vi "review.vi"() -> ()   [LabVIEW 2014]
panel:
  out "클러스터 2":T1
  in  "클러스터":T1
  in  "배열":dbl[](array[numeric])
  out "웨이브폼 차트 2":dbl(graph)
  out "웨이브폼 차트":dbl(graph)
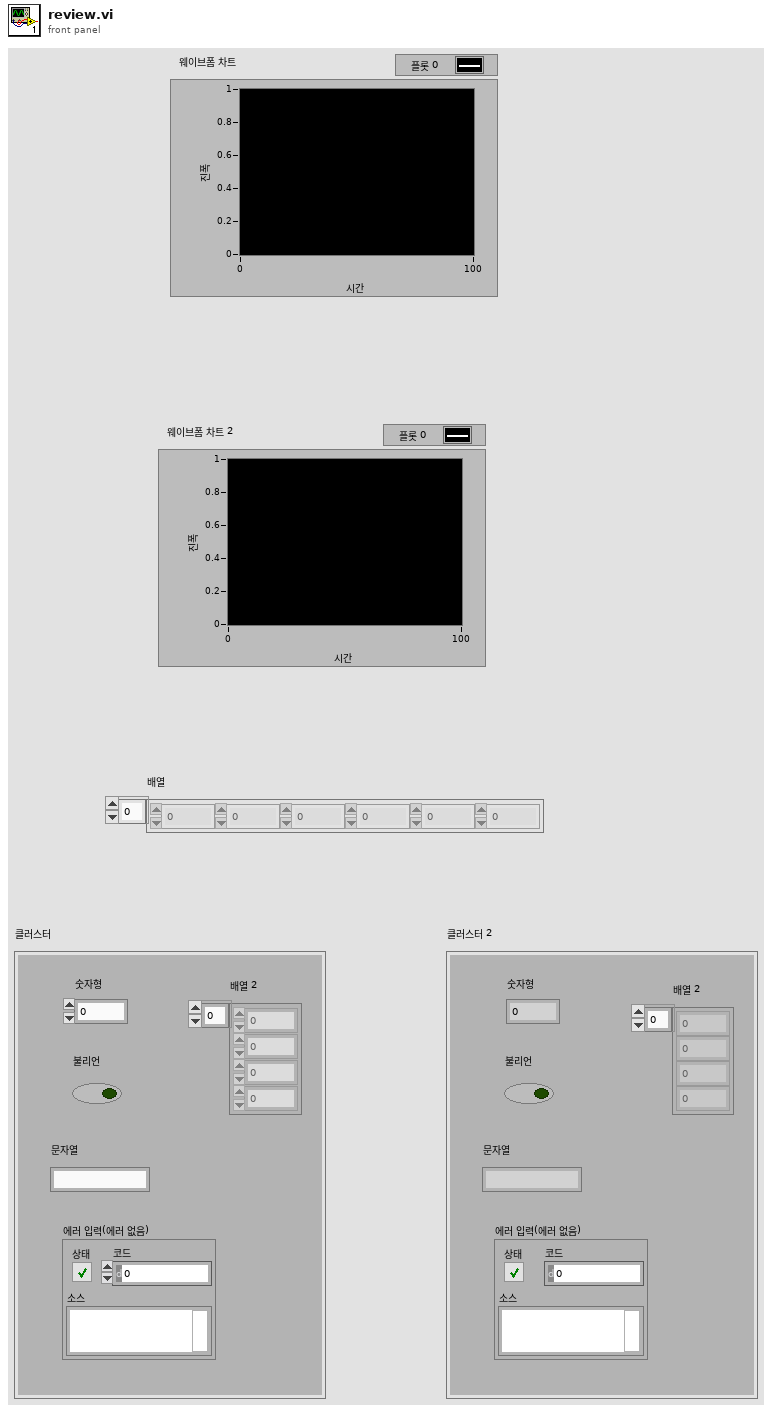
[diagram p1: front panel]
types:
  T1 = cluster{"숫자형":dbl, "불리언":bool, "문자열":string, "배열 2":dbl[], "error in (no error)":errorcluster}
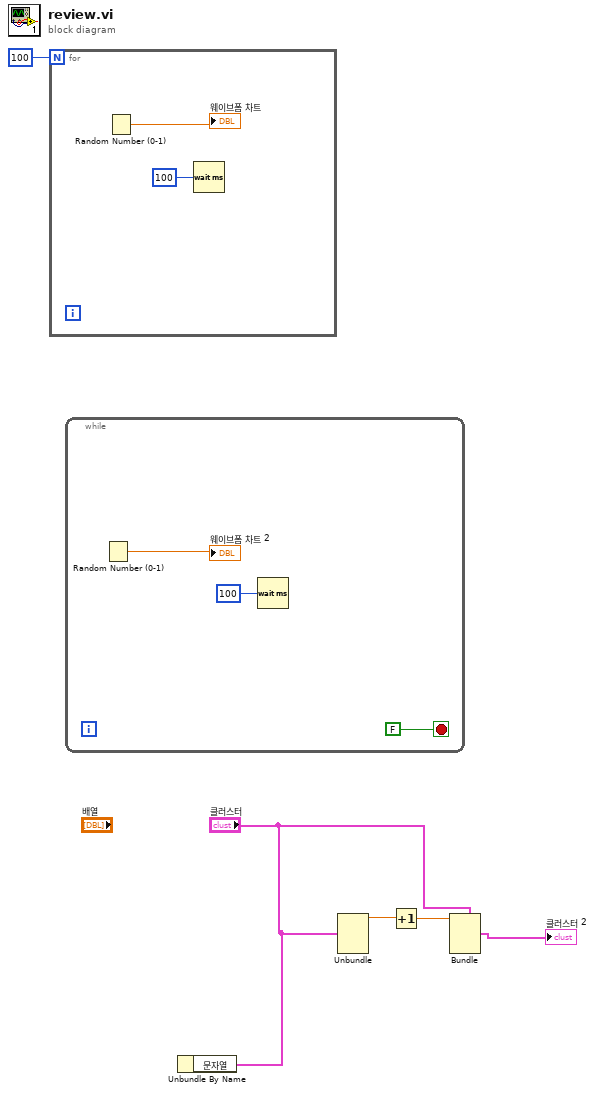
[diagram p0: block diagram]
diagram:
  n1 = for {
    N: 100 -> [_]
    n2 = Random Number (0-1)() -> (number: 0 to 1=→"웨이브폼 차트":dbl)
    n3 = Wait (ms)(milliseconds to wait=u32 100 ("대기 시간(ms)")) -> ()  [unwired: 1 out]
  }
  n4 = while {
    stop <- FALSE stop-if-true
    n5 = Random Number (0-1)() -> (number: 0 to 1=→"웨이브폼 차트 2":dbl)
    n6 = Wait (ms)(milliseconds to wait=u32 100 ("대기 시간(ms)")) -> ()  [unwired: 1 out]
  }
  n7 = Unbundle By Name("클러스터") -> ()  [unwired: 1 out]
  n8 = Unbundle("클러스터") -> ("숫자형"=w2:dbl)  [unwired: 4 out]
  n9 = Increment(x=w2) -> (x+1=w1:dbl)
  n10 = Bundle(cluster="클러스터", "숫자형"=w1) -> (→"클러스터 2":T1)  [unwired: 4 in]
